vi "Write Run Minimized.vi"(8 "error in (no error)":errorcluster, 10 "Run Minimized":bool, 11 "CallEXEStep in":refnum<class "CallEXEStep.lvclass">) -> (0 "error out":errorcluster, 3 "CallEXEStep out":refnum<class "CallEXEStep.lvclass">)   [LabVIEW 2015, in "CallEXEStep.lvclass"]
uses:
  CallEXEStep.lvclass
  CallEXEStep.lvclass/CallEXEStep.ctl
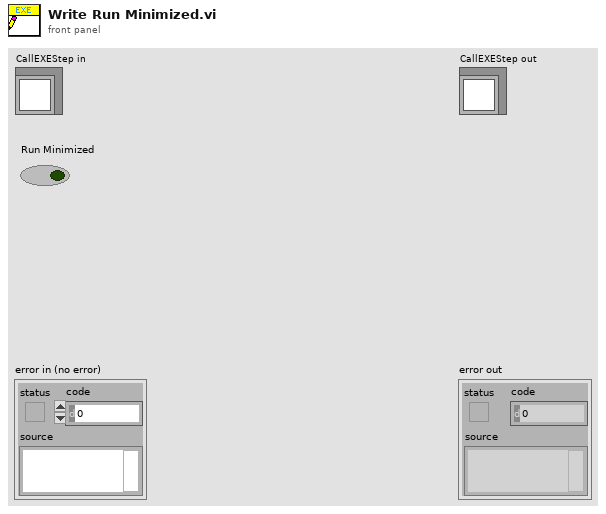
[diagram p1: front panel]
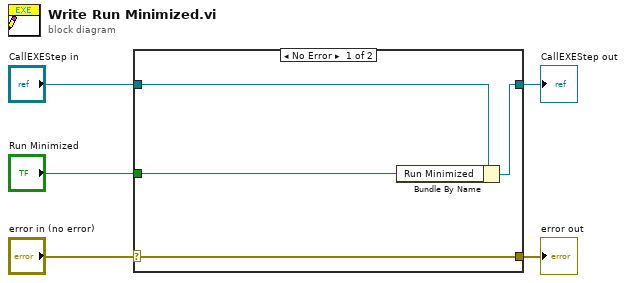
[diagram p0: block diagram]
diagram:
  n1 = case shown="No Error" "error in (no error)" {
    selector: "error in (no error)" -> [w9 w10]
    tunnel: [w9 w10] -> w4
    tunnel: [w7 w11] -> w2
    tunnel: "CallEXEStep in" -> [w8 w11]
    tunnel: "Run Minimized" -> [w6 _]
    frame No Error {
      n2 = Bundle By Name(cluster=w8, "Run Minimized"=w6) -> (w7:refnum<class "CallEXEStep.lvclass">)
    }
    frame Error {
    }
  }
  "error out" <- w4
  "CallEXEStep out" <- w2
